vi "Adaptive Filter.vi"(5 "Beta":fxp<+/-,32,24> format="%.16g", 6 "Element":T2, 9 "Memory In":T1, 11 "Input":i16) -> (3 "Output":i16)   [LabVIEW 2013]
uses:
  Filter Data Blocks.ctl
panel:
  out "Memory Out":T1
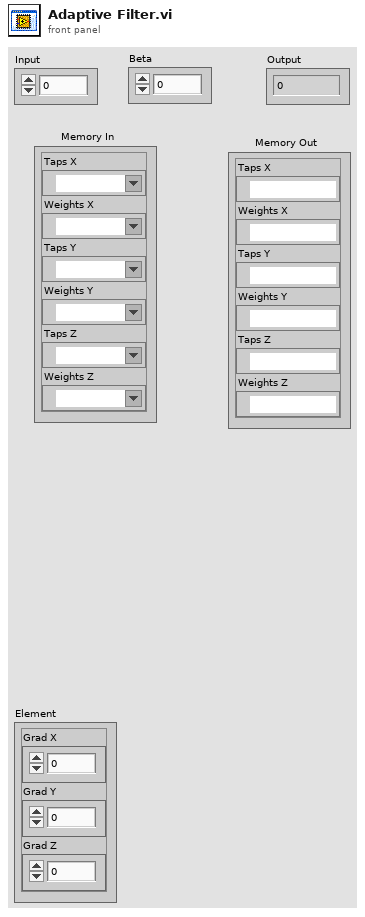
[diagram p1: front panel]
types:
  T1 = typedef "Filter Data Blocks.ctl" = cluster{"Taps X":refnum<k21>, "Weights X":refnum<k21>, "Taps Y":refnum<k21>, "Weights Y":refnum<k21>, "Taps Z":refnum<k21>, "Weights Z":refnum<k21>}
  T2 = cluster{"Grad X":i16, "Grad Y":i16, "Grad Z":i16}
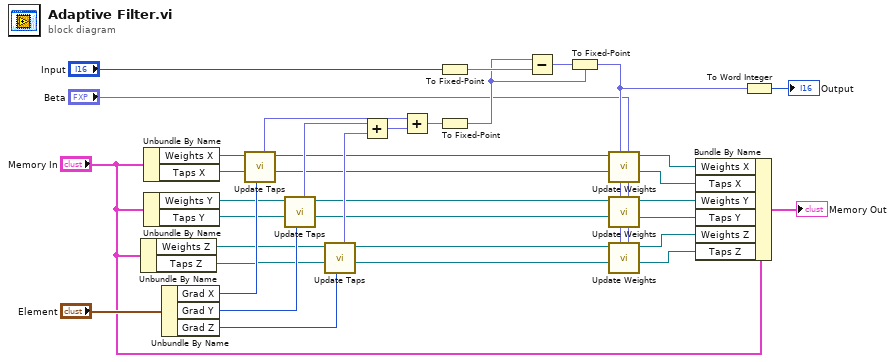
[diagram p0: block diagram]
diagram:
  n1 = Unbundle By Name("Memory In") -> ("Weights Z"=w24:refnum<k21>, "Taps Z"=w23:refnum<k21>)
  n2 = Unbundle By Name("Memory In") -> ("Weights X"=w30:refnum<k21>, "Taps X"=w29:refnum<k21>)
  n3 = Unbundle By Name("Memory In") -> ("Weights Y"=w27:refnum<k21>, "Taps Y"=w26:refnum<k21>)
  n4 = Unbundle By Name("Element") -> ("Grad X"=w28:i16, "Grad Y"=w25:i16, "Grad Z"=w22:i16)
  n5 = call "Update Taps.vi"("Gradient"=w28, "Taps"=w29, "Weights"=w30) -> ("Taps Out"=w16:refnum<k21>, "Weights Out"=w17:refnum<k21>, "FIR Out"=w21:fxp<+/-,32,24>)  [unwired: 6 in]
  n6 = call "Update Taps.vi"("Gradient"=w25, "Taps"=w26, "Weights"=w27) -> ("Taps Out"=w13:refnum<k21>, "Weights Out"=w14:refnum<k21>, "FIR Out"=w20:fxp<+/-,32,24>)  [unwired: 6 in]
  n7 = call "Update Taps.vi"("Gradient"=w22, "Taps"=w23, "Weights"=w24) -> ("Taps Out"=w11:refnum<k21>, "Weights Out"=w12:refnum<k21>, "FIR Out"=w19:fxp<+/-,32,24>)  [unwired: 6 in]
  n8 = Add(x=w20, y=w19) -> (x+y=w18:fxp<+/-,33,25>)
  n9 = Add(x=w21, y=w18) -> (x+y=w31:fxp<+/-,34,26>)
  n10 = To Fixed-Point(number="Input") -> (fixed-point=w32:fxp<+/-,16,16>)  [unwired: 1 in]
  n11 = To Fixed-Point(number=w31) -> (fixed-point=w15:fxp<+/-,32,24>)  [unwired: 1 in]
  n12 = Subtract(x=w15, y=w32) -> (x-y=w33:fxp<+/-,33,25>)
  n13 = To Fixed-Point(fixed-point type=w15, number=w33) -> (fixed-point=w10:fxp<+/-,32,24>)
  n14 = call "Update Weights.vi"("Beta"="Beta", "Error In"=w10, "Taps"=w16, "Weights"=w17) -> ("Taps Out"=w4:refnum<k21>, "Weights Out"=w7:refnum<k21>)  [unwired: 6 in]
  n15 = call "Update Weights.vi"("Beta"="Beta", "Error In"=w10, "Taps"=w13, "Weights"=w14) -> ("Taps Out"=w5:refnum<k21>, "Weights Out"=w6:refnum<k21>)  [unwired: 6 in]
  n16 = call "Update Weights.vi"("Beta"="Beta", "Error In"=w10, "Taps"=w11, "Weights"=w12) -> ("Taps Out"=w2:refnum<k21>, "Weights Out"=w3:refnum<k21>)  [unwired: 6 in]
  n17 = Bundle By Name(cluster="Memory In", "Weights X"=w7, "Taps X"=w4, "Weights Y"=w6, "Taps Y"=w5, "Weights Z"=w3, "Taps Z"=w2) -> (→"Memory Out":T1)
  n18 = To Word Integer(number=w10) -> (16bit integer=→"Output":i16)
